vi "replace error gen.vi"() -> ()   [LabVIEW 2014]
uses:
  <vilib>/Utility/traverseref.llb/TRef TravTarget.ctl
  <vilib>/Utility/traverseref.llb/VI Scripting - Traverse.lvlib
panel:
  in  "new error gen path":path=path "C:/Program Files (x86)/National Instruments/LabVIEW 2013/vi.lib/NI/Configuration Framework/error generator/NISE_error generator.vi"
  in  "old error gen path":path=path "C:/Program Files (x86)/National Instruments/LabVIEW 2013/vi.lib/NI/Configuration Framework/error generator.vi"
  in  "Path":path
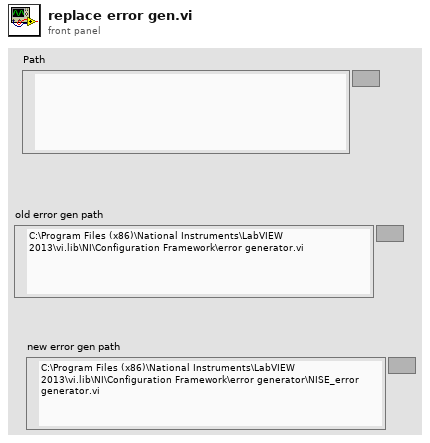
[diagram p1: front panel]
types:
  T1 = typedef "TRef TravTarget.ctl" = enum16{"FP", "BD", "Other"}
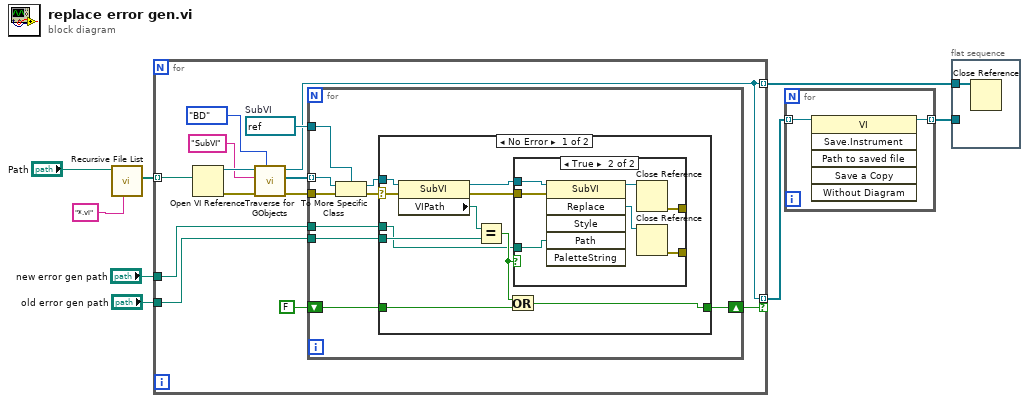
[diagram p0: block diagram]
diagram:
  n1 = call <vilib>:"Recursive File List.vi"("pattern"="*.vi", "Folder Path"="Path") -> ("All Files in Dir"=w6:path[])  [unwired: 5 in, 4 out]
  n2 = for {
    tunnel: w6 -> [w21] mode=indexing
    tunnel: [w13] -> w3 mode=indexing
    tunnel: [w13] -> w5 mode=indexing if=w12
    tunnel: "old error gen path" -> [w11]
    tunnel: "new error gen path" -> [w10]
    w16 = refnum<vi> refnum  # SubVI
    n3 = Open VI Reference(vi path=w21) -> (vi reference=w20:refnum<vi>, error out=w19:errorcluster)  [unwired: 5 in]
    n4 = call <vilib>:"Traverse for GObjects.vi"("Traverse Target"=TRef_TravTarget."BD", "error in (no error)"=w19, "Class Name"="SubVI", "VI Refnum"=w20) -> ("error out"=w15:errorcluster, "References"=w17:refnum<vi>[], "dup VI Refnum"=w13:refnum<vi>)  [unwired: 4 in, 1 out]
    n5 = for {
      tunnel: w17 -> [w30] mode=indexing
      tunnel: w16 -> [w29]
      tunnel: w15 -> [w28]
      shift-right: [w24] -> w12
      shift-left: FALSE -> [w25]
      tunnel: w11 -> [w23]
      tunnel: w10 -> [w22]
      n6 = To More Specific Class(target class=w29, reference=w30, error in=w28) -> (specific class reference=w26:refnum<vi>, error out=w27:errorcluster)
      n7 = case shown="No Error" w27 {
        selector: w27 -> [w40 _]
        tunnel: w26 -> [w39 _]
        tunnel: w25 -> [w35 w48]
        tunnel: [w36 w48] -> w24
        tunnel: w23 -> [w37 _]
        tunnel: w22 -> [w31 _]
        frame No Error {
          n8 = property class="SubVI"(reference=w39, error in=w40) -> (reference out=w33:refnum<vi>, error out=w32:errorcluster, "VIPath"=w38:path)
          n9 = Equal?(x=w38, y=w37) -> (x = y?=w34:bool)
          n10 = Or(x=w34, y=w35) -> (x .or. y?=w36:bool)
          n11 = case shown="True" w34 {
            tunnel: w33 -> [_ w47]
            tunnel: w32 -> [_ w46]
            tunnel: [_ w43] -> _
            tunnel: [_ w42] -> _
            tunnel: w31 -> [_ w41]
            frame False {
            }
            frame True {
              n12 = invoke class="SubVI" method="Replace"(reference=w47, error in=w46, "Path"=w41) -> (reference out=w45:refnum<vi>, "Replace"=w44:refnum<vi>)  [unwired: 3 in, 4 out]
              n13 = Close Reference(reference=w45) -> (error out=w42:errorcluster)  [unwired: 1 in]
              n14 = Close Reference(reference=w44) -> (error out=w43:errorcluster)  [unwired: 1 in]
            }
          }
        }
        frame Error {
        }
      }
    }
  }
  n15 = for {
    tunnel: w5 -> [w50] mode=indexing
    tunnel: [w49] -> w4 mode=indexing
    n16 = invoke class="VI" method="Save.Instrument"(reference=w50) -> (reference out=w49:refnum<vi>)  [unwired: 5 in, 5 out]
  }
  n17 = flat-sequence {
    tunnel: w4 -> [_]
    tunnel: w3 -> [w51]
    frame #0 {
      n18 = Close Reference(reference=w51) -> ()  [unwired: 1 in, 1 out]
    }
  }
